vi "Test Error Handler Interface Handle Warnings.vi"(8 "error in (no error)":errorcluster, 11 "Test Case In":refnum<class "Error Handler Interface Test.lvclass">) -> (0 "error out":errorcluster, 3 "Test Case Out":refnum<class "Error Handler Interface Test.lvclass">)   [LabVIEW 2020, in "Error Handler Interface Test.lvclass"]
uses:
  Error Handler Interface Test.lvclass
  C:/Program Files (x86)/National Instruments/LabVIEW 2020/vi.lib/Asteme/LUnit/Test Case.lvclass
  Error Handler Interface Test.lvclass/Error Handler Interface Test.ctl
  <vilib>/Asteme/LUnit/Test Case.lvclass/Test Case.ctl
  <vilib>/Asteme/LUnit/LUnit Assertion Result.lvclass/LUnit Assertion Result.ctl
  <vilib>/Asteme/LUnit/Palette/Pass.vi
  <vilib>/Asteme/LUnit/Palette/Fail.vi
  <vilib>/Asteme/LUnit/Variant to string.vi
  <vilib>/Asteme/LUnit/Set Assertion Type.vi
  <vilib>/Asteme/LUnit/Add test result.vi
  <vilib>/Asteme/LUnit/LUnit Write Passed.vi
  <vilib>/Asteme/LUnit/LUnit Get Test Case.vi
  <vilib>/Asteme/LUnit/LUnit Write Message.vi
  <vilib>/Asteme/LUnit/LUnit Write Description.vi
  <vilib>/Asteme/LUnit/LUnit Write Assertion Type.vi
  <vilib>/Asteme/LUnit/Read Test Case Name.vi
  <vilib>/Asteme/LUnit/Assertion Result/LUnit Get Test Name.vi
  <vilib>/Utility/Data Type/Get Type Information.vi
  <vilib>/Utility/LVClass/Get LV Class Name.vi
  Framework/Error Handler Interface/Error Handler Interface.lvclass
  <vilib>/Asteme/LUnit/LUnit Assertion Result.lvclass
  <vilib>/Asteme/LUnit/Test Case.lvclass
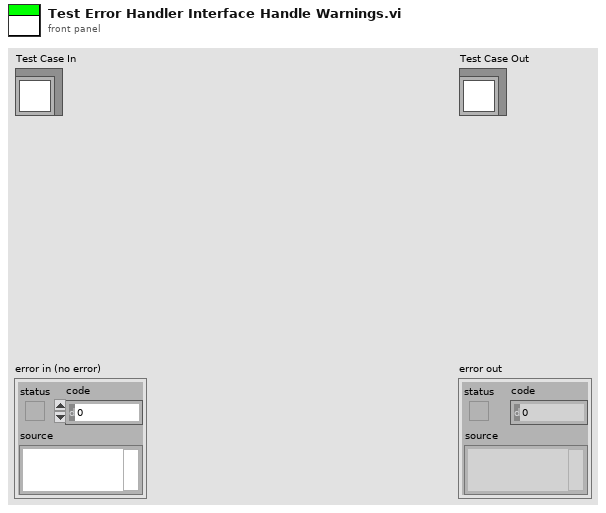
[diagram p1: front panel]
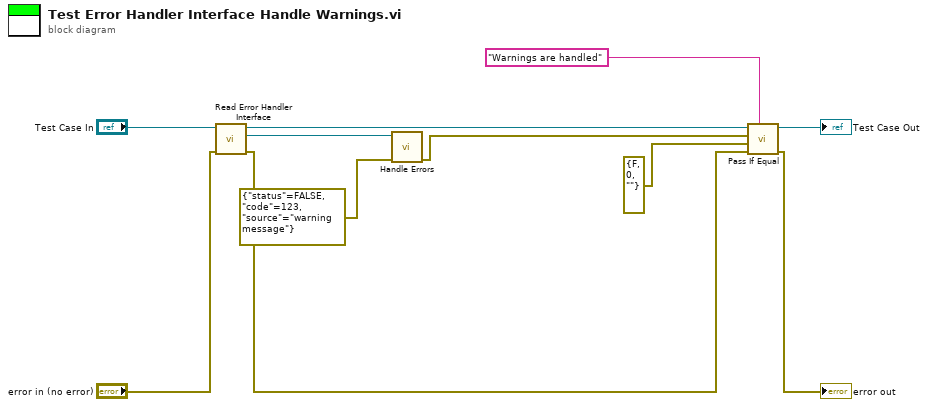
[diagram p0: block diagram]
diagram:
  n1 = call "Read Error Handler Interface.vi"("error in (no error)"="error in (no error)", "Error Handler Interface Test in"="Test Case In") -> ("error out"=w3:errorcluster, "Error Handler Interface"=w8:refnum<class "Error Handler Interface.lvclass">, "Error Handler Interface Test out"=w9:refnum<class "Error Handler Interface Test.lvclass">)  [unwired: 7 in]
  n2 = call-dynamic "Handle Errors.vi"("error in (no error)"=errorcluster {"status"=FALSE, "code"=123, "source"="warning message"}, "Error Handler Interface In"=w8) -> ("error out"=w5:errorcluster)  [unwired: 8 in, 1 out]
  n3 = call <vilib>:"Pass If Equal.vi"("Description"="Warnings are handled", "error in (no error)"=w3, "Actual"=errorcluster {"status"=FALSE, "code"=0, "source"=""} ("error out"), "Expected"=w5, "Test Case In"=w9) -> ("error out"=→"error out":errorcluster, "Test Case Out"=→"Test Case Out":refnum<class "Error Handler Interface Test.lvclass">)  [unwired: 5 in]
